vi "02secuencia_equipos.vi"(0 "Paneles in":T2(array[cluster]) {"Numeric" min=1.0 max=60.0 step=1.0 format="%#2.1f"; "Ultima recepción" format="%<%d/%m - %X>T"; "Med\nPpal" format="%_4g"}, 1 "dif eq?":bool, 2 "ver equipo":i32(ring) caption="TELECOMANDAR EQUIPO N°" items=["1", "2", "3", "4", "5", "6", "7", "8", "9", "10", "11", "12", "13", "14", "15", "16", "17", "18", "19", "20", "21", "22", "23", "24", "25"], 3 "Eq unico":bool caption="Prioridad\nUnica de equipo", 4 "Config Equipos":T1(array[cluster])=[{"Modelo"="", "IP"="", "Puerto"=0, "Time Out"=0, "Med Princ"=0, "Time sin rx"=60, "Reintento"=60, "Ref PD"=200}] {"Ref PD" max=10000 step=1; "Med Princ" items=["1", "2", "3", "4", "5", "6", "7", "8", "9", "10", "11", "12", "13", "14", "15", "16", "17", "18", "19", "20", "21", "22", "23", "24", "25", "26", "27", "28", "29", "30", "31", "32"]}) -> (5 "Secuencia hab":T3(array[cluster]))   [LabVIEW 2010]
panel:
  in  "Flags \nreintento":bool[](array[boolean])
  out "T. desc":timestamp[](array[timestamp])
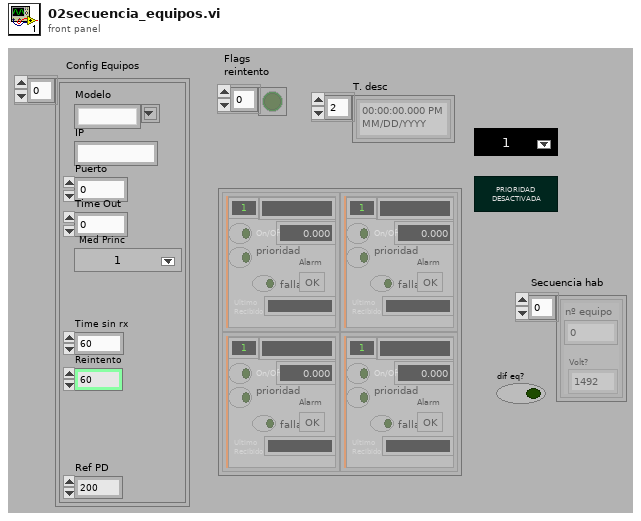
[diagram p1: front panel]
types:
  T1 = cluster{"Modelo":string, "IP":string, "Puerto":u16, "Time Out":u16, "Med Princ":u16, "Time sin rx":u16, "Reintento":u16, "Ref PD":u16}[]
  T2 = cluster{"Nombre":string, "Med\nPpal":dbl, "On/Off":bool, "Ultima recepción":timestamp, "Numeric":dbl, "STOP 2":bool, "prioridad":bool, "falla":bool, "Alarm":bool}[][]
  T3 = cluster{"nº equipo":i32, "Volt?":enum32{"492", "1492", "307", "568", "1568"}}[]
  T4 = cluster{"Modelo":string, "IP":string, "Puerto":u16, "Time Out":u16, "Med Princ":u16, "Time sin rx":u16, "Reintento":u16, "Ref PD":u16}
  T5 = cluster{"Nombre":string, "Med\nprinc":dbl, "On/Off":bool, "Ultima recepción":timestamp, "Nº":dbl, "deshabilitacion":bool, "Actividad":bool, "falla":bool, "alarm":bool}
  T6 = cluster{i32, "Volt?":enum32{"492", "1492", "307", "568", "1568"}}
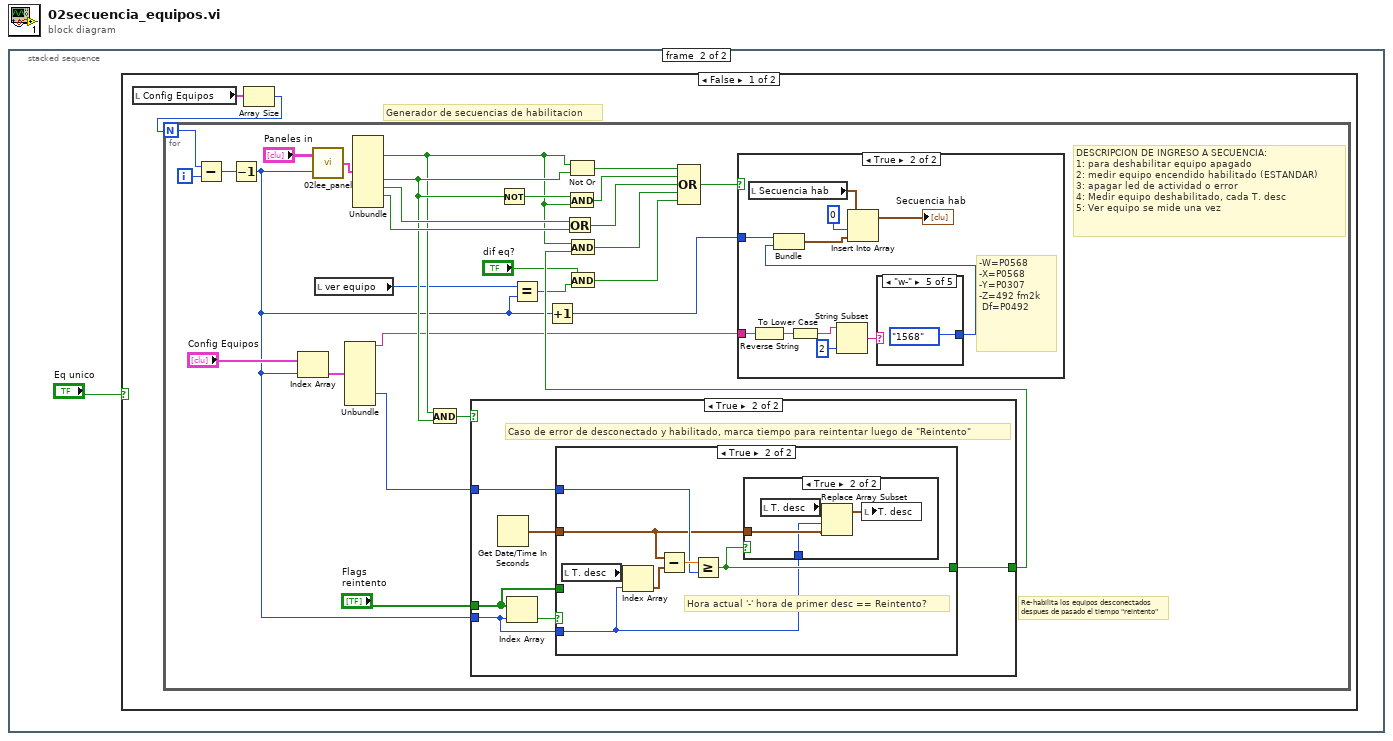
[diagram p0: block diagram]
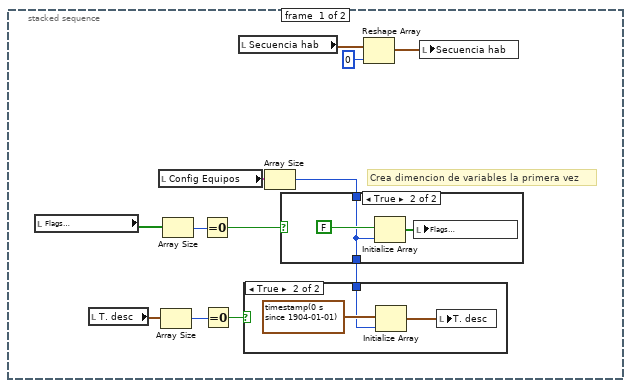
[diagram p2: hidden frame]
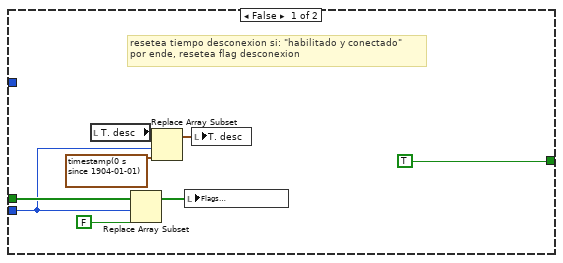
[diagram p5: hidden frame]
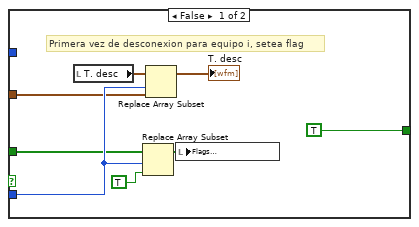
[diagram p6: hidden frame]
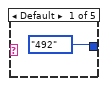
[diagram p9: hidden frame]
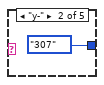
[diagram p10: hidden frame]
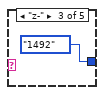
[diagram p11: hidden frame]
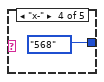
[diagram p12: hidden frame]
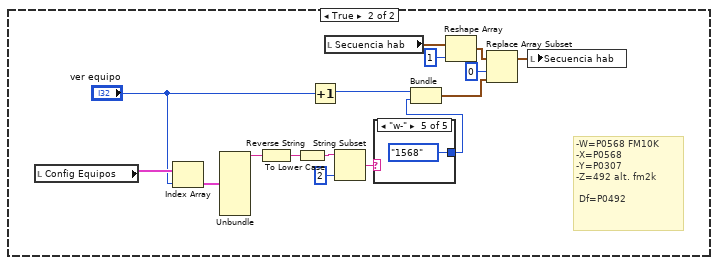
[diagram p13: hidden frame]
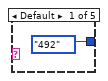
[diagram p14: hidden frame]
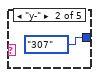
[diagram p15: hidden frame]
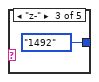
[diagram p16: hidden frame]
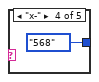
[diagram p17: hidden frame]
diagram:
  n1 = stacked-sequence {
    frame #0 {
      # "Crea dimencion de variables la primera vez"
      n2 = local read "Flags \nreintento"() -> (w9:bool[])
      n3 = local read "T. desc"() -> (w8:timestamp[])
      n4 = local read "Config Equipos"() -> (w2:T1)
      n5 = Array Size(array=w8) -> (size(s)=w4:i32)
      n6 = Array Size(array=w9) -> (size(s)=w7:i32)
      n7 = Equal To 0?(x=w7) -> (x = 0?=w6:bool)
      n8 = Equal To 0?(x=w4) -> (x = 0?=w5:bool)
      n9 = local read "Secuencia hab"() -> (w10:T3)
      n10 = Array Size(array=w2) -> (size(s)=w1:i32)
      n11 = case shown="True" w6 {
        tunnel: w1 -> [w16 w17]
        tunnel: [w16 w17] -> w3
        frame False {
        }
        frame True {
          n12 = Initialize Array(FALSE, w17) -> (w19:bool[])
          n13 = local write "Flags \nreintento"(w19) -> ()
        }
      }
      n14 = case shown="True" w5 {
        tunnel: w3 -> [_ w13]
        frame False {
        }
        frame True {
          n15 = Initialize Array(timestamp(0 s since 1904-01-01), w13) -> (w15:timestamp[])
          n16 = local write "T. desc"(w15) -> ()
        }
      }
      n17 = Reshape Array(w10, 0 ("dimension size")) -> (w11:T3)
      n18 = local write "Secuencia hab"(w11) -> ()
    }
    frame #1 {
      n19 = case shown="False" "Eq unico" {
        frame False {
          # "Generador de secuencias de habilitacion"
          n20 = local read "Config Equipos"() -> (w22:T1)
          n21 = Array Size(array=w22) -> (size(s)=w21:i32)
          n22 = for {
            N: w21 -> [w50]
            i -> [w32]
            # "DESCRIPCION DE INGRESO A SECUENCIA:\n1: para deshabilitar equipo apagado\n2: medir equipo encendido habilitado (ESTANDAR)\n3: apagar led de actividad o error\n4: Medir equipo deshabilitado, cada T. desc\n5: Ver equipo se mide una vez"
            # "Re-habilita los equipos desconectados\ndespues de pasado el tiempo \"reintento\""
            n23 = Subtract(x=w50, y=w32) -> (x-y=w30:i32)
            n24 = Decrement(x=w30) -> (x-1=w28:i32)
            n25 = Index Array(array="Config Equipos", index=w28) -> (element=w49:T4)
            n26 = call "02lee_panel.vi"("Equipo Nº"=w28, "Paneles"="Paneles in") -> ("Panel"=w48:T5)
            n27 = local read "ver equipo"() -> (w24:i32)
            n28 = Unbundle(w49) -> ("Modelo"=w31:string, "Reintento"=w39:u16)  [unwired: 6 out]
            n29 = Unbundle(w48) -> ("On/Off"=w33:bool, "deshabilitacion"=w35:bool, "Actividad"=w38:bool, "falla"=w37:bool)  [unwired: 5 out]
            n30 = And(x=w33, y=w35) -> (x .and. y?=w34:bool)
            n31 = case shown="True" w34 {
              tunnel: w28 -> [w51 w63]
              tunnel: w39 -> [_ w62]
              tunnel: "Flags \nreintento" -> [w56 w61]
              tunnel: [TRUE ("new element/subarray") w60] -> w40
              frame False {
                # "resetea tiempo desconexion si: \"habilitado y conectado\"\npor ende, resetea flag desconexion"
                n32 = local read "T. desc"() -> (w53:timestamp[])
                n33 = Replace Array Subset(array=w56, new element=FALSE ("new element/subarray"), index=w51) -> (w58:bool[])
                n34 = Replace Array Subset(array=w53, new element=timestamp(0 s since 1904-01-01) ("new element/subarray"), index=w51) -> (w52:timestamp[])
                n35 = local write "Flags \nreintento"(w58) -> ()
                n36 = local write "T. desc"(w52) -> ()
              }
              frame True {
                # "Caso de error de desconectado y habilitado, marca tiempo para reintentar luego de \"Reintento\""
                n37 = Get Date/Time In Seconds() -> (seconds since 1Jan1904=w59:timestamp)
                n38 = Index Array(array=w61, index=w63) -> (element=w64:bool)
                n39 = case shown="True" w64 {
                  tunnel: w63 -> [w68 w73]
                  tunnel: w61 -> [w67 _]
                  tunnel: w62 -> [_ w76]
                  tunnel: [TRUE w74] -> w60
                  tunnel: w59 -> [w65 w75]
                  frame False {
                    # "Primera vez de desconexion para equipo i, setea flag"
                    n40 = local read "T. desc"() -> (w72:timestamp[])
                    n41 = Replace Array Subset(array=w67, new element=TRUE ("new element/subarray"), index=w68) -> (w70:bool[])
                    n42 = Replace Array Subset(array=w72, new element=w65, index=w68) -> (→"T. desc":timestamp[])
                    n43 = local write "Flags \nreintento"(w70) -> ()
                  }
                  frame True {
                    # "Hora actual '-' hora de primer desc == Reintento?"
                    n44 = local read "T. desc"() -> (w79:timestamp[])
                    n45 = Index Array(array=w79, index=w73) -> (element=w78:timestamp)
                    n46 = Subtract(x=w75, y=w78) -> (x-y=w77:dbl)
                    n47 = Greater Or Equal?(x=w77, y=w76) -> (x >= y?=w74:bool)
                    n48 = case shown="True" w74 {
                      tunnel: w75 -> [_ w81]
                      tunnel: w73 -> [_ w80]
                      frame False {
                      }
                      frame True {
                        n49 = local read "T. desc"() -> (w83:timestamp[])
                        n50 = Replace Array Subset(array=w83, new element=w81, index=w80) -> (w82:timestamp[])
                        n51 = local write "T. desc"(w82) -> ()
                      }
                    }
                  }
                }
              }
            }
            n52 = Not(x=w35) -> (.not. x?=w42:bool)
            n53 = Equal?(x=w24, y=w28) -> (x = y?=w25:bool)
            n54 = Increment(x=w28) -> (x+1=w29:i32)
            n55 = Or(x=w38, y=w37) -> (x .or. y?=w36:bool)
            n56 = Not Or(1:w35, 2:w33) -> (0:w43:bool)
            n57 = And(x=w42, y=w33) -> (x .and. y?=w41:bool)
            n58 = And(x=w33, y=w40) -> (x .and. y?=w27:bool)
            n59 = And(x="dif eq?", y=w25) -> (x .and. y?=w26:bool)
            n60 = Compound Arithmetic op=OR(w43, w41, w36, w27, w26) -> (w44:bool)
            n61 = case shown="True" w44 {
              tunnel: w29 -> [_ w87]
              tunnel: w31 -> [_ w93]
              frame False {
              }
              frame True {
                # "-W=P0568\n-X=P0568\n-Y=P0307\n-Z=492 fm2k\n Df=P0492"
                n62 = local read "Secuencia hab"() -> (w94:T3)
                n63 = Reverse String(1:w93) -> (0:w92:string)
                n64 = To Lower Case(string=w92) -> (all lower case string=w89:string)
                n65 = String Subset(string=w89, length (rest)=2 ("length (rest)")) -> (substring=w86:string)  [unwired: 1 in]
                n66 = case shown="\"w-\"" w86 {
                  tunnel: [enum32{"492", "492B", "307", "568"}."492" ("Volt?") enum32{"492", "492B", "307", "568"}."307" ("Volt?") enum32{"492", "1492", "307", "568"}."1492" ("Volt?") enum32{"492", "492B", "307", "568"}."568" ("Volt?") enum32{"492", "492B", "307", "568", "1568"}."1568" ("Volt?")] -> w85
                  frame Default {
                  }
                  frame "y-" {
                  }
                  frame "z-" {
                  }
                  frame "x-" {
                  }
                  frame "w-" {
                  }
                }
                n67 = Bundle(w87, "Volt?"=w85) -> (w84:cluster{i32, "Volt?":u32})  [unwired: 1 in]
                n68 = Insert Into Array(array=w94, index=0, new element=w84) -> (→"Secuencia hab":T3)
              }
            }
          }
        }
        frame True {
          # "-W=P0568 FM10K\n-X=P0568\n-Y=P0307\n-Z=492 alt. fm2k\n\n Df=P0492"
          n69 = local read "Config Equipos"() -> (w110:T1)
          n70 = Index Array(array=w110, index="ver equipo") -> (element=w109:T4)
          n71 = Unbundle(w109) -> ("Modelo"=w102:string)  [unwired: 7 out]
          n72 = Reverse String(1:w102) -> (0:w107:string)
          n73 = To Lower Case(string=w107) -> (all lower case string=w106:string)
          n74 = Increment(x="ver equipo") -> (x+1=w103:i32)
          n75 = local read "Secuencia hab"() -> (w115:T3)
          n76 = String Subset(string=w106, length (rest)=2 ("length (rest)")) -> (substring=w104:string)  [unwired: 1 in]
          n77 = case shown="\"w-\"" w104 {
            tunnel: [enum32{"492", "1492", "307", "568"}."492" ("Volt?") enum32{"492", "1492", "307", "568"}."307" ("Volt?") enum32{"492", "1492", "307", "568"}."1492" ("Volt?") enum32{"492", "1492", "307", "568"}."568" ("Volt?") enum32{"492", "1492", "307", "568", "1568"}."1568" ("Volt?")] -> w100
            frame Default {
            }
            frame "y-" {
            }
            frame "z-" {
            }
            frame "x-" {
            }
            frame "w-" {
            }
          }
          n78 = Bundle(w103, "Volt?"=w100) -> (w101:T6)  [unwired: 1 in]
          n79 = Reshape Array(w115, 1 ("dimension size")) -> (w112:T3)
          n80 = Replace Array Subset(array=w112, new element=w101, index=0) -> (w111:T3)
          n81 = local write "Secuencia hab"(w111) -> ()
        }
      }
    }
  }
